vi "Start_DAQ_and_stim.vi"(6 "error in":errorcluster, 7 "All frontpanel parameters":T1 {"Free run parameters"."Stim length" min=0.001 max=0.1 step=0.01; "Free run parameters"."Stim onset" min=0.0 max=100.0; "Free run parameters"."Stim frequency" min=0.1 max=40.0 step=1.0; "Device parameters"."Read chunk size" min=100 max=100000; "Device parameters"."Acquisition sample rate" min=10.0 max=10000.0 step=10.0; "Device parameters"."Stimulation sample rate" min=10.0 max=10000.0; "Protocol parameters"."Pulse width" min=0.0001 max=0.1 step=0.01; "Protocol parameters"."Acquire after ON" min=0.0 max=10.0 step=1.0; "Protocol parameters"."Acquire before ON" min=0.0 max=10.0 step=1.0; "Protocol parameters"."Repetitions" min=1.0 max=10.0 step=1.0; "Protocol parameters"."OFF time" min=0.0 max=1000.0; "Protocol parameters"."ON time" min=0.0 max=1000.0; "Protocol parameters"."Stim onset" min=0.0 max=100.0; "Protocol parameters"."Stim frequency" min=0.1 max=40.0 step=1.0}, 8 "Control_Stim_Queue":refnum<queue>, 9 "Control_DAQ_Queue":refnum<queue>) -> (0 "error out":errorcluster)   [LabVIEW 2010]
uses:
  typedefs/control_stim_enum.ctl
  typedefs/all_frontpanel_parameters_protocol_NI.ctl
  typedefs/run_mode.ctl
  typedefs/protocol_parameters.ctl
  typedefs/free_run_parameters.ctl
  typedefs/device_parameters.ctl
  typedefs/storage_parameters_cluster.ctl
  typedefs/control_daq_enum.ctl
panel:
  # "_0000.txt"
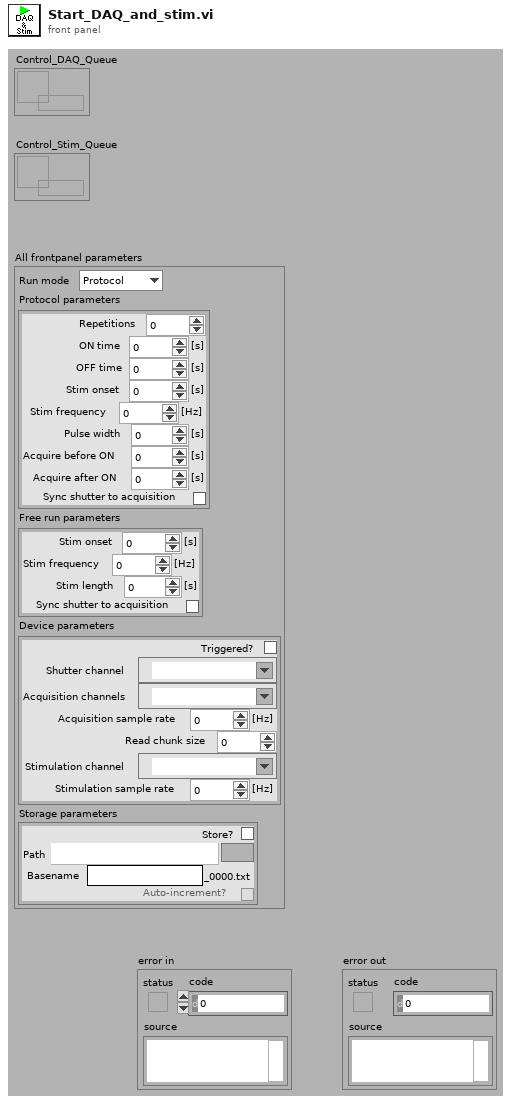
[diagram p1: front panel]
types:
  T1 = typedef "all_frontpanel_parameters_protocol_NI.ctl" = cluster{"Run mode":T2, "Protocol parameters":T3, "Free run parameters":T4, "Device parameters":T5, "Storage parameters":T6}
  T2 = typedef "run_mode.ctl" = enum32{"Protocol", "Free Run"}
  T3 = typedef "protocol_parameters.ctl" = cluster{"Repetitions":dbl, "ON time":dbl, "OFF time":dbl, "Stim onset":dbl, "Stim frequency":dbl, "Pulse width":dbl, "Acquire before ON":dbl, "Acquire after ON":dbl, "Sync shutter to acquisition":bool}
  T4 = typedef "free_run_parameters.ctl" = cluster{"Stim onset":dbl, "Stim frequency":dbl, "Stim length":dbl, "Sync shutter to acquisition":bool}
  T5 = typedef "device_parameters.ctl" = cluster{"Triggered?":bool, "Shutter channel":tag, "Acquisition channels":tag, "Acquisition sample rate":dbl, "Read chunk size":i32, "Stimulation channel":tag, "Stimulation sample rate":dbl}
  T6 = typedef "storage_parameters_cluster.ctl" = cluster{"Store?":bool, "Path":path, "Basename":string, "Auto-increment?":bool}
  T7 = typedef "control_stim_enum.ctl" = enum16{"Init", "Stim Protocol", "Stim Free Run", "Stop", "Quit"}
  T8 = typedef "control_daq_enum.ctl" = enum16{"Init", "FreeRun", "Protocol", "Stop", "Quit"}
  T9 = cluster{"Device parameters":T5, "Protocol parameters":T3}
  T10 = cluster{"Device parameters":T5, "Free run parameters":T4}
  T11 = cluster{"Control stim Enum":T7, "Variant":variant}
  T12 = cluster{"Control DAQ Enum":T8, "Variant":variant}
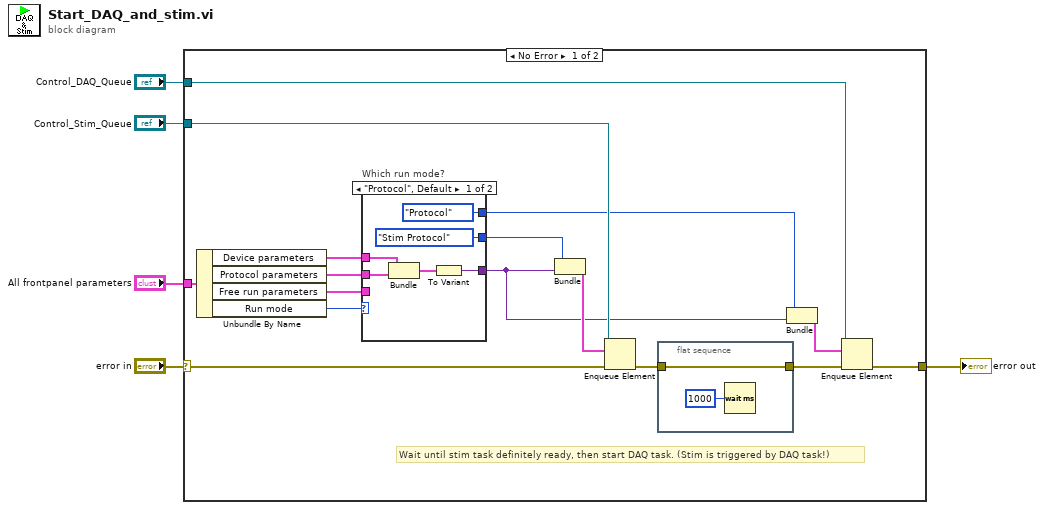
[diagram p0: block diagram]
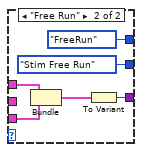
[diagram p2: hidden frame]
diagram:
  n1 = case shown="No Error" "error in" {
    selector: "error in" -> [w13 w36]
    tunnel: "Control_Stim_Queue" -> [w18 _]
    tunnel: "All frontpanel parameters" -> [w17 _]
    tunnel: [w16 w36] -> w3
    tunnel: "Control_DAQ_Queue" -> [w15 _]
    frame No Error {
      # "Wait until stim task definitely ready, then start DAQ task. (Stim is triggered by DAQ task!)"
      n2 = Unbundle By Name(w17) -> ("Device parameters"=w12:T5, "Protocol parameters"=w10:T3, "Free run parameters"=w9:T4, "Run mode"=w11:T2)
      n3 = case "Which run mode?" shown="\"Protocol\", Default" w11 {
        tunnel: w12 -> [w27 w33]
        tunnel: w10 -> [w26 _]
        tunnel: w9 -> [_ w32]
        tunnel: [w24 w30] -> w8
        tunnel: [control_daq_enum."Protocol" ("Control DAQ Enum") control_daq_enum."FreeRun" ("Control DAQ Enum")] -> w7
        tunnel: [control_stim_enum."Stim Protocol" ("Control stim Enum") control_stim_enum."Stim Free Run" ("Control stim Enum")] -> w6
        frame "Protocol", Default {
          n4 = Bundle("Device parameters"=w27, "Protocol parameters"=w26) -> (w25:T9)  [unwired: 1 in]
          n5 = To Variant(anything=w25) -> (Variant=w24:variant)
        }
        frame "Free Run" {
          n6 = Bundle("Device parameters"=w33, "Free run parameters"=w32) -> (w31:T10)  [unwired: 1 in]
          n7 = To Variant(anything=w31) -> (Variant=w30:variant)
        }
      }
      n8 = Bundle("Control stim Enum"=w6, "Variant"=w8) -> (w19:T11)  [unwired: 1 in]
      n9 = Enqueue Element(queue=w18, element=w19, error in (no error)=w13) -> (error out=w20:errorcluster)  [unwired: 1 in, 2 out]
      n10 = flat-sequence {
        tunnel: w20 -> [w35]
        tunnel: [w35] -> w21
        frame #0 {
          n11 = Wait (ms)(milliseconds to wait=u32 1000) -> ()  [unwired: 1 out]
        }
      }
      n12 = Bundle("Control DAQ Enum"=w7, "Variant"=w8) -> (w14:T12)  [unwired: 1 in]
      n13 = Enqueue Element(queue=w15, element=w14, error in (no error)=w21) -> (error out=w16:errorcluster)  [unwired: 1 in, 2 out]
    }
    frame Error {
    }
  }
  "error out" <- w3
